vi "Get Public Events.vi"(8 "error in (no error)":errorcluster, 11 "JKI_Python_Server in":refnum<class "Server.lvclass">) -> (0 "error out":errorcluster, 2 "Public Events":T1, 3 "JKI_Python_Server out":refnum<class "Server.lvclass">)   [LabVIEW 2013, in "JKI_Python_Bridge_for_LV.lvlib" / "Server.lvclass"]
uses:
  Server.lvclass
  Type Definitions/Public Events - Cluster.ctl
  Server.lvclass/Server.ctl
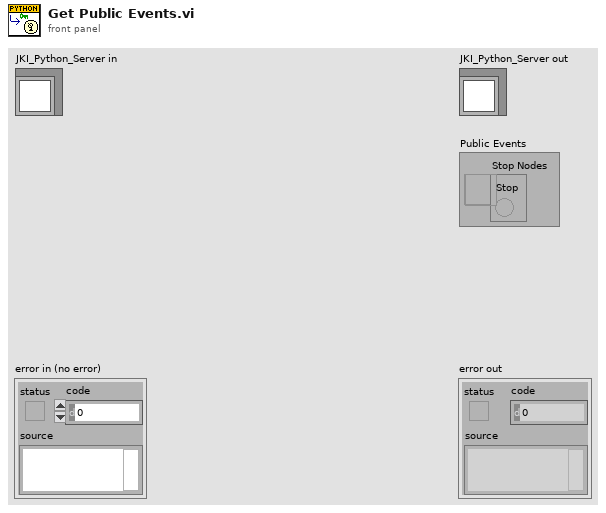
[diagram p1: front panel]
types:
  T1 = typedef "JKI_Python_Bridge_for_LV.lvlib/Server.lvclass/Public Events - Cluster.ctl" = cluster{"Stop Nodes":refnum<user-event>}
  T2 = typedef "JKI_Python_Bridge_for_LV.lvlib/Server.lvclass/Class Private Data - Cluster.ctl" = cluster{"TCP Server RefNum":T3, "TCP port (50007)":u16, "max connections (0: no limit)":u32, "net address (0: Listen on All Adaptors)":u32, "Nodes":T4[], "Public Events":T1}
  T3 = typedef "TCP Server Object RefNum__jki_lib_tcp_server.ctl" = refnum<k1>
  T4 = typedef "JKI_Python_Bridge_for_LV.lvlib/Server.lvclass/Python Node.ctl" = cluster{"Name":string, "Python Method Call":refnum<user-event>, "Call Handle":refnum<class "CallHandler.lvclass">}
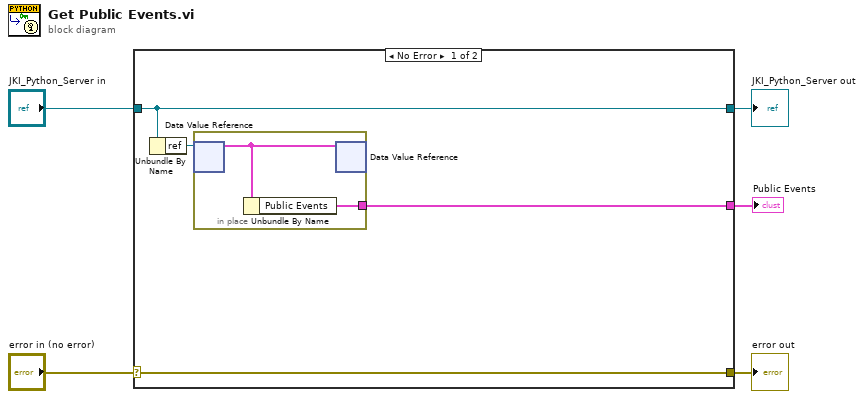
[diagram p0: block diagram]
diagram:
  n1 = case shown="No Error" "error in (no error)" {
    selector: "error in (no error)" -> [w7 w13]
    tunnel: [w7 w13] -> w4
    tunnel: [w9 w12] -> w2
    tunnel: "JKI_Python_Server in" -> [w9 w12]
    tunnel: [w6 _] -> w1
    frame No Error {
      n2 = Unbundle By Name(w9) -> ("ref"=w8:refnum<data-value>)
      n3 = in-place {
        in-place-border: [w10] -> w6
        n4 = in-place-dvr #1(w8) -> (w11:T2)  [unwired: 1 out]
        n5 = Unbundle By Name(w11) -> ("Public Events"=w10:T1)
        n6 = in-place-dvr #1(w11) -> ()  [unwired: 2 out]
      }
    }
    frame Error {
    }
  }
  "error out" <- w4
  "JKI_Python_Server out" <- w2
  "Public Events" <- w1
